vi "[Teste]GraphWrite.vi"() -> ()   [LabVIEW 2014]
panel:
  in  "stop":bool
  out "Numeric":dbl
  out "Waveform Chart":dbl(graph)
  in  "Escolha: Porta Serial":refnum<visa-resource-name>="COM3"
  out "String":string
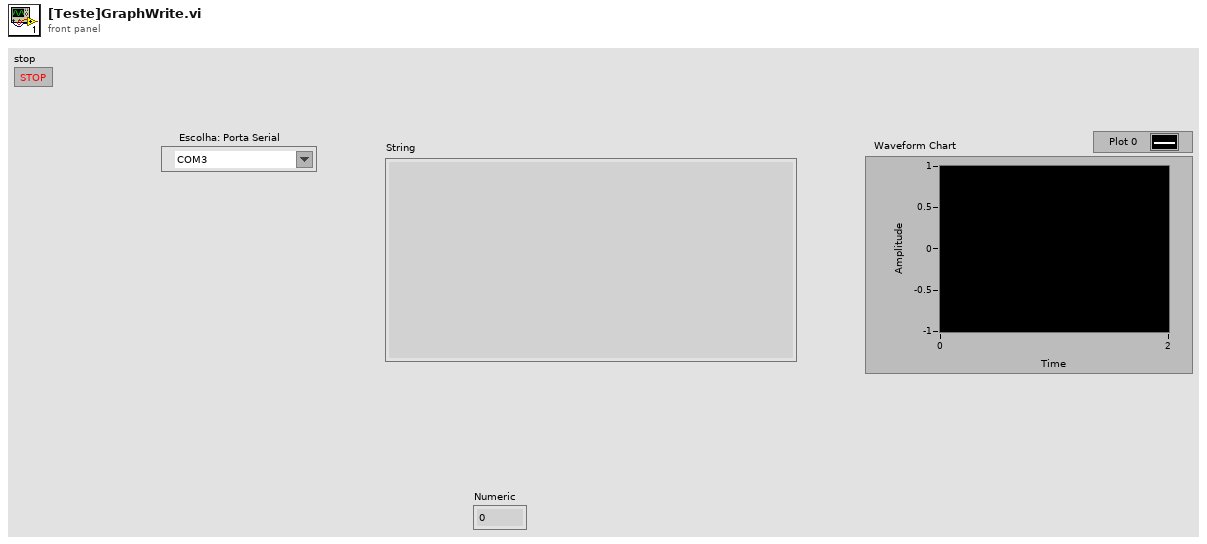
[diagram p1: front panel]
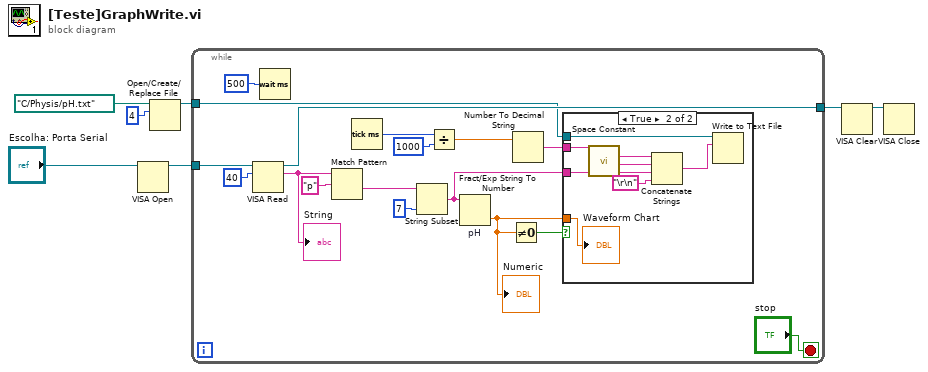
[diagram p0: block diagram]
diagram:
  n1 = VISA Open(VISA resource name="Escolha: Porta Serial") -> (VISA resource name=w6:refnum<visa-resource-name>)  [unwired: 4 in, 1 out]
  n2 = Open/Create/Replace File(file path (use dialog)=path "C:/Physis/pH.txt", operation (0:open)=4) -> (refnum out=w1:refnum<file>)  [unwired: 4 in, 2 out]
  n3 = while {
    tunnel: w6 -> [w23]
    tunnel: [w20] -> w4
    tunnel: w1 -> [w9]
    stop <- "stop" stop-if-true
    n4 = VISA Read(VISA resource name=w23, byte count=40) -> (VISA resource name out=w20:refnum<visa-resource-name>, read buffer=w18:string)  [unwired: 1 in, 2 out]
    "String" <- w18
    n5 = Wait (ms)(milliseconds to wait=500) -> ()  [unwired: 1 out]
    n6 = Match Pattern(string=w18, regular expression="p") -> (after substring=w17:string)  [unwired: 1 in, 3 out]
    n7 = Tick Count (ms)() -> (millisecond timer value=w13:u32)
    n8 = String Subset(string=w17, length (rest)=7) -> (substring=w10:string)  [unwired: 1 in]
    n9 = Divide(x=w13, y=1000) -> (x/y=w12:dbl)
    n10 = Fract/Exp String To Number "pH"(string=w10) -> (number=w15:dbl)  [unwired: 3 in, 1 out]
    "Numeric" <- w15
    n11 = Not Equal To 0?(x=w15) -> (x != 0?=w16:bool)
    n12 = Number To Decimal String(number=w12) -> (decimal integer string=w11:string)  [unwired: 1 in]
    n13 = case shown="True" w16 {
      tunnel: w15 -> [_ w31]
      tunnel: w11 -> [_ w30]
      tunnel: w10 -> [_ w28]
      tunnel: w9 -> [_ w26]
      frame False {
      }
      frame True {
        n14 = call <vilib>:"Space Constant.vi"() -> ("String"=w29:string)
        n15 = Concatenate Strings(w30, w29, w28, "\r\n") -> (w27:string)
        n16 = Write to Text File(file (use dialog)=w26, text=w27) -> ()  [unwired: 2 in, 3 out]
        "Waveform Chart" <- w31
      }
    }
  }
  n17 = VISA Clear(VISA resource name=w4) -> (VISA resource name out=w5:refnum<visa-resource-name>)  [unwired: 1 in, 1 out]
  n18 = VISA Close(VISA resource name=w5) -> ()  [unwired: 1 in, 1 out]
